vi "SR430_get_records_per_scan.vi"(0 "address":T1, 5 "error in (no error)":errorcluster) -> (14 "addressOut":T1, 16 "recordsPerScan":i32, 19 "error out":errorcluster)   [LabVIEW 2009, in "SR430Driver.lvlib"]
doc: "reads the number of records per scan (set-value).\n\nThe \"records per scan\" must be between 0 <= i <= 65535\n\nIf records per scan equals 0, accumulation will continue indefinitely.\n\nCopyright (C)\nGesellschaft für Schwerionenforschung, GSI\nPlanckstr. 1\n64291 Darmstadt\nGermany\n\nContact: D.Beck@gsi.de \n\nThis program is free software; you can redistribute it and/or modify it under the terms of the \nGNU General Public License as published by the Free Software Foundation; either version 2 of the license, or (at your option) any later version.\n\nThis program is distributed in the hope that it will be useful, but WITHOUT ANY WARRANTY; without even the implied warranty of MERCHANTABILITY or FITNESS FOR A PARTICULAR PURPOSE. See the GNU General License for more details (http://www.gnu.org).\n\nGesellschaft für Schwerionenforschung, GSI\nPlanckstr. 1, 64291 Darmstadt, Germany\nFor all questions and ideas contact: M.Richter@gsi.de, K.Poppensieker, H.Brand@gsi.de or D.Beck@gsi.de.\nLast update: 11-APR-2002"
uses:
  SR430Driver.lvlib
  SR430_VISA Control.ctl
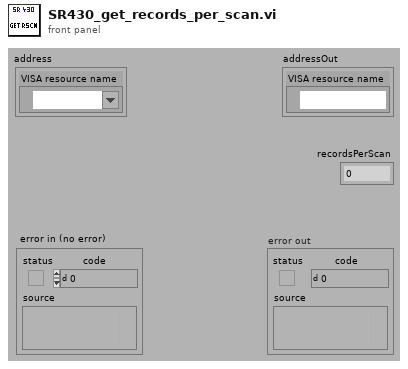
[diagram p1: front panel]
types:
  T1 = typedef "SR430Driver.lvlib/SR430_VISA Control.ctl" = cluster{"VISA resource name":refnum<visa-resource-name>}
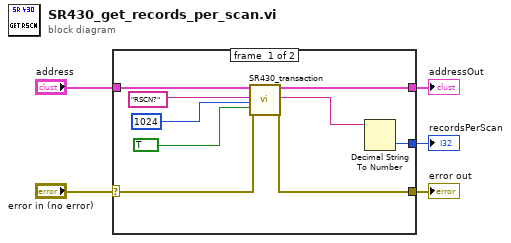
[diagram p0: block diagram]
diagram:
  n1 = case shown="No Error" "error in (no error)" {
    selector: "error in (no error)" -> [w12 w16]
    tunnel: [w14 _] -> w5
    tunnel: [w11 w16] -> w4
    tunnel: "address" -> [w13 w15]
    tunnel: [w10 w15] -> w2
    frame #0 {
      n2 = call "SR430_transaction.vi"("SR430 VISA Cluster"=w13, "SR430 Command String"="RSCN?" ("write buffer"), "Bytes to read (1024)"=u32 1024, "Read (FALSE)"=TRUE, "error in (no error)"=w12) -> ("dup SR430 VISA Cluster"=w10:T1, "SR430 Response"=w9:string, "error out"=w11:errorcluster)  [unwired: 11 in, 1 out]
      n3 = Decimal String To Number(string=w9) -> (number=w14:i32)  [unwired: 2 in, 1 out]
    }
    frame #1 {
    }
  }
  "addressOut" <- w2
  "error out" <- w4
  "recordsPerScan" <- w5
